vi "gate_controller.vi"(10 "Numerical Argument":dbl, 11 "Command":T1(ring)=enum."Read Voltage") -> (3 "Response":string)   [LabVIEW 2021]
panel:
  # "GATE CONTROLLER"
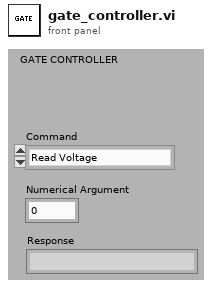
[diagram p1: front panel]
types:
  T1 = enum16{"Set Voltage", "Read Voltage", "Read Current", "Output On", "Output Off", "Set Increment", "Set Increment Time", "Stop Voltage Set", "Set Maximum Voltage", "Get Maximum Voltage"}
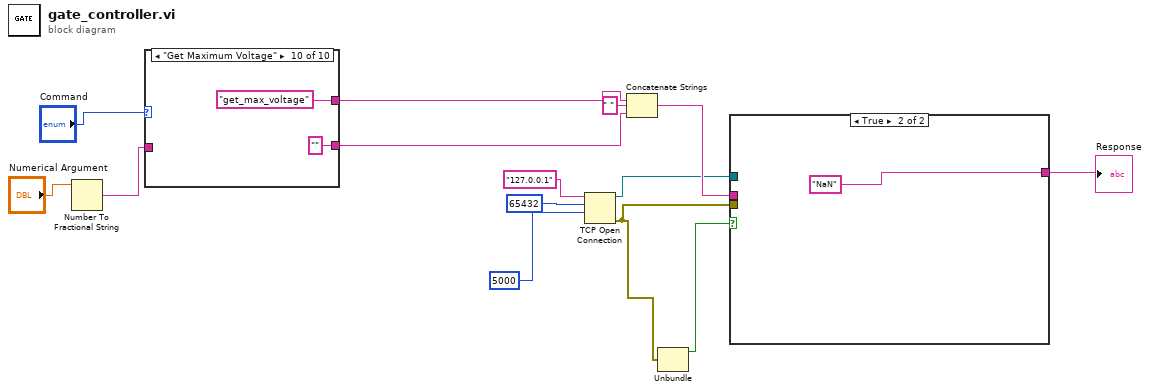
[diagram p0: block diagram]
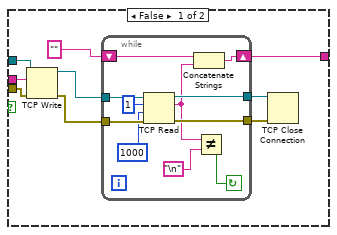
[diagram p2: hidden frame]
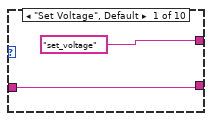
[diagram p3: hidden frame]
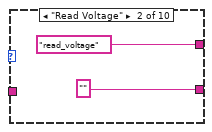
[diagram p4: hidden frame]
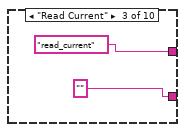
[diagram p5: hidden frame]
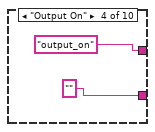
[diagram p6: hidden frame]
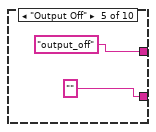
[diagram p7: hidden frame]
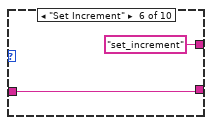
[diagram p8: hidden frame]
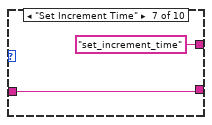
[diagram p9: hidden frame]
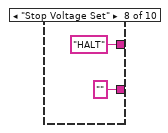
[diagram p10: hidden frame]
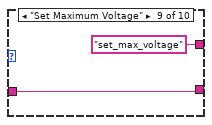
[diagram p11: hidden frame]
diagram:
  n1 = Number To Fractional String(number="Numerical Argument") -> (F-format string=w8:string)  [unwired: 3 in]
  n2 = case shown="\"Get Maximum Voltage\"" "Command" {
    tunnel: ["set_voltage" ("data in") "read_voltage" ("data in") "read_current" ("data in") "output_on" ("data in") "output_off" ("data in") "set_increment" ("data in") "set_increment_time" ("data in") "HALT" ("data in") "set_max_voltage" ("data in") "get_max_voltage" ("data in")] -> w12
    tunnel: [w15 "" ("string") "" ("string") "" ("string") "" ("string") w26 w28 "" ("string") w32 "" ("string")] -> w9
    tunnel: w8 -> [w15 _ _ _ _ w26 w28 _ w32 _]
    frame "Set Voltage", Default {
    }
    frame "Read Voltage" {
    }
    frame "Read Current" {
    }
    frame "Output On" {
    }
    frame "Output Off" {
    }
    frame "Set Increment" {
    }
    frame "Set Increment Time" {
    }
    frame "Stop Voltage Set" {
    }
    frame "Set Maximum Voltage" {
    }
    frame "Get Maximum Voltage" {
    }
  }
  n3 = TCP Open Connection(address="127.0.0.1", remote port or service name=u16 65432, timeout ms (60000)=5000) -> (connection ID=w1:refnum<k5>, error out=w3:errorcluster)  [unwired: 2 in]
  n4 = Concatenate Strings(w12, " " ("string"), w9) -> (w2:string)
  n5 = Unbundle(w3) -> ("status"=w4:bool)  [unwired: 2 out]
  n6 = case shown="True" w4 {
    tunnel: [w40 "NaN"] -> w5
    tunnel: w3 -> [w39 _]
    tunnel: w2 -> [w38 _]
    tunnel: w1 -> [w37 _]
    frame False {
      n7 = TCP Write(connection ID=w37, data in=w38, error in (no error)=w39) -> (connection ID out=w35:refnum<k5>, error out=w36:errorcluster)  [unwired: 1 in, 1 out]
      n8 = while {
        tunnel: w36 -> [w54]
        tunnel: w35 -> [w53]
        tunnel: [w52] -> w43
        tunnel: [w51] -> w42
        shift-right: [w47] -> w40
        shift-left: "" ("string") -> [w48]
        stop <- w46 continue-if-true
        n9 = TCP Read(connection ID=w53, bytes to read=1, error in (no error)=w54, 9:1000 ("timeout ms (25000)")) -> (connection ID out=w51:refnum<k5>, data out=w45:string, error out=w52:errorcluster)  [unwired: 1 in]
        n10 = Concatenate Strings(w48, w45) -> (w47:string)
        n11 = Not Equal?(x=w45, y="\n") -> (x != y?=w46:bool)
      }
      n12 = TCP Close Connection(connection ID=w42, error in (no error)=w43) -> ()  [unwired: 1 in, 2 out]
    }
    frame True {
    }
  }
  "Response" <- w5
